vi "split arraty.vi"(10 "Datos bruto":string[][](array[string]), 11 "Parametro":string="a") -> (2 "Datos segundo parametro":string[](array[string]), 3 "Datos parametro":string[](array[string]))   [LabVIEW 2018]
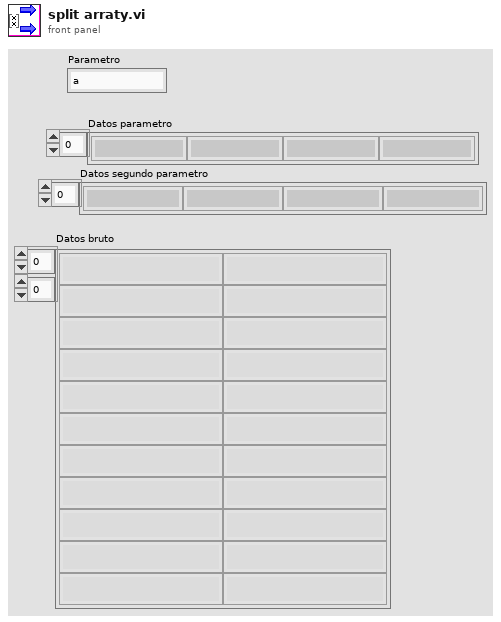
[diagram p1: front panel]
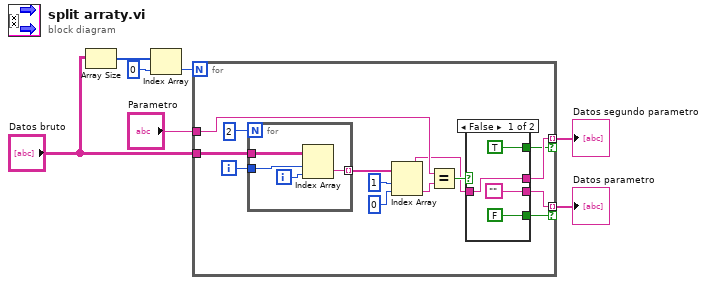
[diagram p0: block diagram]
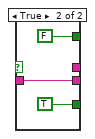
[diagram p2: hidden frame]
diagram:
  n1 = Array Size(array="Datos bruto") -> (size(s)=w5:i32[])
  n2 = Index Array(array=w5, index=0) -> (element=w4:i32)
  n3 = for {
    N: w4 -> [_]
    tunnel: "Datos bruto" -> [w20]
    tunnel: "Parametro" -> [w16]
    tunnel: [w14] -> w1 mode=indexing if=w11
    tunnel: [w13] -> w2 mode=indexing if=w12
    i -> [w21]
    n4 = for {
      N: 2 -> [_]
      tunnel: w21 -> [w32]
      tunnel: w20 -> [w31]
      tunnel: [w29] -> w18 mode=indexing
      i -> [w30]
      n5 = Index Array(array=w31, index (row)=w32, index (col)=w30) -> (element=w29:string)
    }
    n6 = Index Array(array=w18, index #1=1 ("index"), index #2=0 ("index")) -> (element #1=w8:string, element #2=w9:string)
    n7 = Equal?(x=w16, y=w9) -> (x = y?=w15:bool)
    n8 = case shown="False" w15 {
      tunnel: w8 -> [w25 w28]
      tunnel: ["" w28] -> w14
      tunnel: [w25 _] -> w13
      tunnel: [TRUE FALSE] -> w12
      tunnel: [FALSE TRUE] -> w11
      frame False {
      }
      frame True {
      }
    }
  }
  "Datos parametro" <- w1
  "Datos segundo parametro" <- w2
